vi "GetGridDriftCorrection(SubVI).vi"(8 "error in (no error)":errorcluster, 11 "Application in":refnum<vi>) -> (0 "Error out":errorcluster, 1 "Y offset":dbl, 2 "X offset":dbl, 3 "Application ref out":refnum<vi>)   [LabVIEW 2014]
uses:
  <userlib>/Nanonis Prog Interface V5/Scan/Grid/GridPatternGet.vi
  <userlib>/Nanonis Prog Interface V5/Nanonis Prog Interface.lvlib
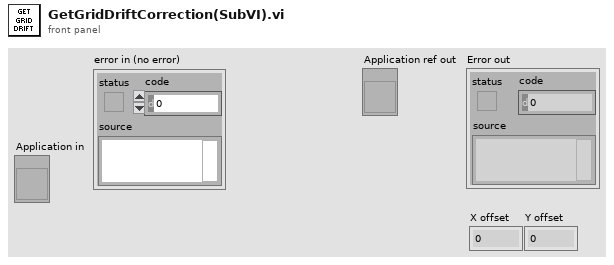
[diagram p1: front panel]
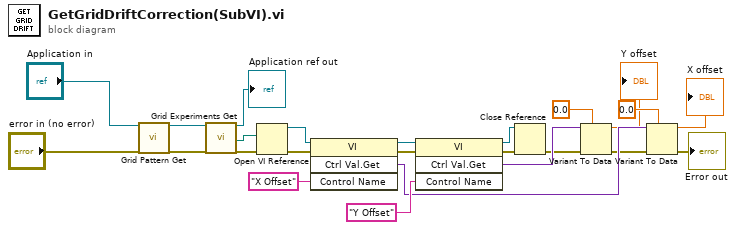
[diagram p0: block diagram]
diagram:
  n1 = call-poly <userlib>:"Grid Pattern Get.vi"("Application ref in"="Application in", "error in (no error)"="error in (no error)") -> ("Application ref out"=w19:refnum<vi>, "error out"=w21:errorcluster)  [unwired: 9 in, 7 out]
  n2 = call <userlib>:"Grid Experiments Get.vi"("Application ref in"=w19, "error in (no error)"=w21) -> ("Application ref out"=→"Application ref out":refnum<vi>, "External VI path"=w24:path, "error out"=w23:errorcluster)  [unwired: 11 in, 4 out]
  n3 = Open VI Reference(vi path=w24, error in (no error)=w23) -> (vi reference=w18:refnum<vi>, error out=w17:errorcluster)  [unwired: 4 in]
  n4 = invoke class="VI" method="Ctrl Val.Get"(reference=w18, error in=w17, "Control Name"="X Offset") -> (reference out=w14:refnum<vi>, error out=w11:errorcluster, "Get Control Value Variant"=w7:variant)  [unwired: 1 in, 1 out]
  n5 = invoke class="VI" method="Ctrl Val.Get"(reference=w14, error in=w11, "Control Name"="Y Offset") -> (reference out=w13:refnum<vi>, error out=w12:errorcluster, "Get Control Value Variant"=w9:variant)  [unwired: 1 in, 1 out]
  n6 = Close Reference(reference=w13, error in (no error)=w12) -> (error out=w5:errorcluster)
  n7 = Variant To Data(error in=w5, type=0.0, Variant=w9) -> (data=→"Y offset":dbl, error out=w4:errorcluster)
  n8 = Variant To Data(error in=w4, type=0.0, Variant=w7) -> (data=→"X offset":dbl, error out=→"Error out":errorcluster)
